vi "flow measure.vi"() -> ()   [LabVIEW 2016]
uses:
  <vilib>/Instr/_visa.llb/VISA Configure Serial Port (Instr).vi
panel:
  out "Flow (L/Min)":string
  out "Flow(L/Min)":dbl(knob) scale=0.0..30.0
  out "Waveform Chart":i32(graph)
  in  "stop":bool
  in  "VISA resource name":refnum<visa-resource-name>
  in  "baud rate (38400)":u32=9600
  # "FLOW  MONITOR"
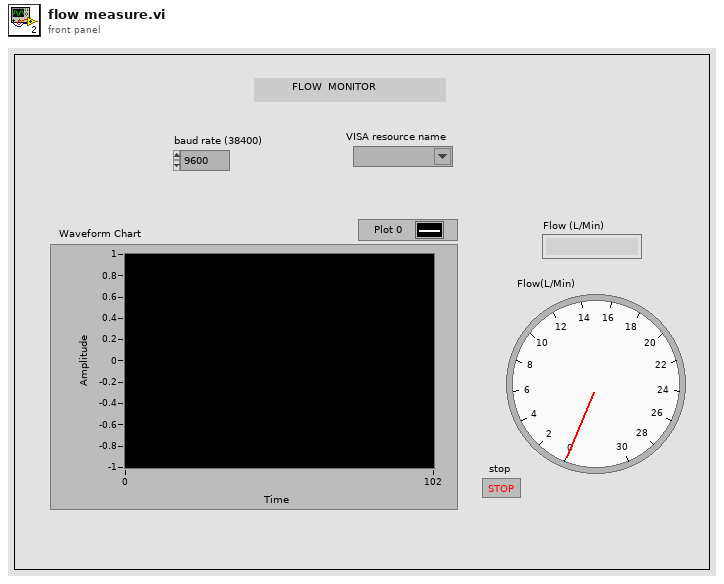
[diagram p1: front panel]
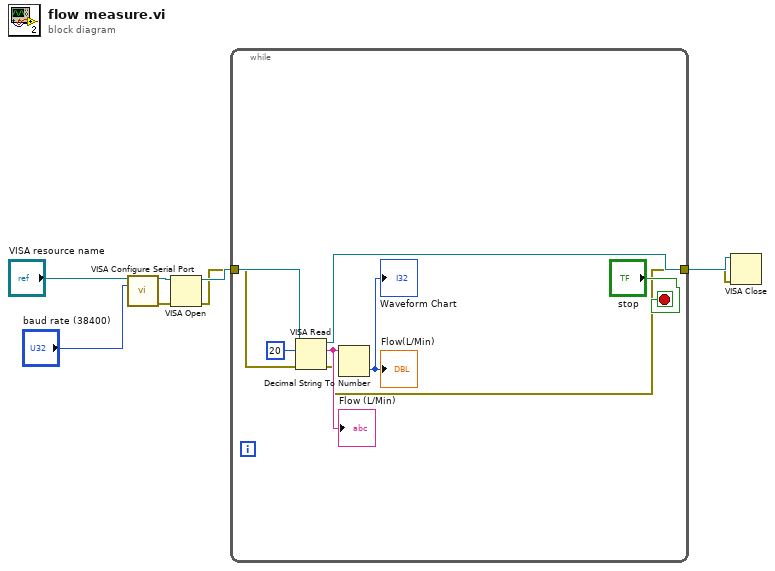
[diagram p0: block diagram]
diagram:
  n1 = call-poly "VISA Configure Serial Port"("VISA resource name"="VISA resource name", "baud rate (9600)"="baud rate (38400)") -> ("VISA resource name out"=w6:refnum<visa-resource-name>, "error out"=w5:errorcluster)  [unwired: 12 in]
  n2 = VISA Open(error in (no error)=w5, VISA resource name=w6) -> (VISA resource name=w4:refnum<visa-resource-name>, error out=w3:errorcluster)  [unwired: 3 in]
  n3 = while {
    tunnel: w4 -> [w16]
    tunnel: w3 -> [w15]
    tunnel: [w11] -> w2
    tunnel: [w10] -> w1
    stop <- "stop" stop-if-true
    n4 = VISA Read(VISA resource name=w16, byte count=u32 20, error in (no error)=w15) -> (VISA resource name out=w11:refnum<visa-resource-name>, read buffer=w12:string, error out=w10:errorcluster)  [unwired: 1 out]
    "Flow (L/Min)" <- w12
    n5 = Decimal String To Number(string=w12) -> (number=→"Waveform Chart" →"Flow(L/Min)":i32)  [unwired: 2 in, 1 out]
  }
  n6 = VISA Close(VISA resource name=w2, error in (no error)=w1) -> ()  [unwired: 1 out]
